vi "Write Display Control.vi"(8 "error in (no error)":errorcluster, 9 "Display Control":T1, 11 "PCF8574 I2C LCD in":refnum<class "PCF8574 I2C LCD.lvclass">) -> (0 "error out":errorcluster, 3 "PCF8574 I2C LCD out":refnum<class "PCF8574 I2C LCD.lvclass">)   [LabVIEW 2020, in "CTI-Peripheral.lvlib" / "PCF8574 I2C LCD.lvclass"]
uses:
  PCF8574 I2C LCD.lvclass
  HD44780 LCD/Display Control.ctl
  HD44780 LCD/Command.ctl
  PCF8574 I2C LCD.lvclass/PCF8574 I2C LCD.ctl
  HD44780 LCD/HD44780 LCD.lvlib
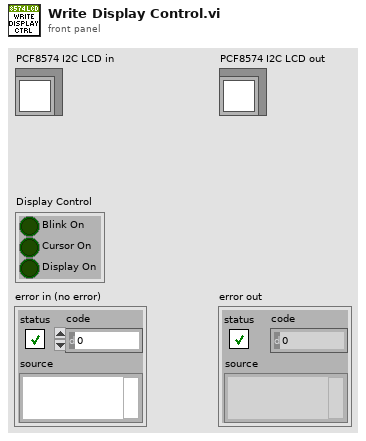
[diagram p1: front panel]
types:
  T1 = typedef "CTI-Peripheral.lvlib/HD44780 LCD.lvlib/Display Control.ctl" = cluster{"Blink On":bool, "Cursor On":bool, "Display On":bool}
  T2 = typedef "CTI-Peripheral.lvlib/HD44780 LCD.lvlib/Command.ctl" = enum16{"ClearDisplay", "ReturnHome", "EntryModeSet", "DisplayControl", "CursorShift", "FunctionSet", "SetCGRamAddr", "SetDDRamAddr"}
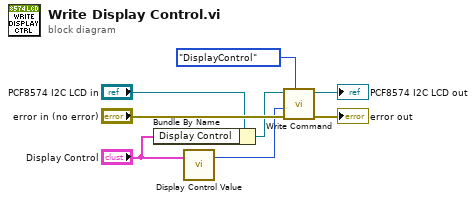
[diagram p0: block diagram]
diagram:
  n1 = Bundle By Name(cluster="PCF8574 I2C LCD in", "Display Control"="Display Control") -> (w5:refnum<class "PCF8574 I2C LCD.lvclass">)
  n2 = call "Display Control Value.vi"("Display Control"="Display Control") -> ("DCtrl Value"=w2:u8)  [unwired: 6 in]
  n3 = call "Write Command.vi"("Command"=Command."DisplayControl", "error in (no error)"="error in (no error)", "Value (0)"=w2, "PCF8574 I2C LCD in"=w5) -> ("error out"=→"error out":errorcluster, "PCF8574 I2C LCD out"=→"PCF8574 I2C LCD out":refnum<class "PCF8574 I2C LCD.lvclass">)  [unwired: 6 in]
